vi "LoadGame.vi"(8 "error in (no error)":errorcluster, 10 "NewGame":refnum<class "Game.lvclass">, 11 "Engine in":refnum<class "Engine.lvclass">) -> (0 "error out":errorcluster, 3 "Engine out":refnum<class "Engine.lvclass">)   [LabVIEW 2019, in "RT_Game.lvlib" / "Engine.lvclass"]
uses:
  Engine.lvclass
  Game/Game.lvclass
  Engine.lvclass/Engine.ctl
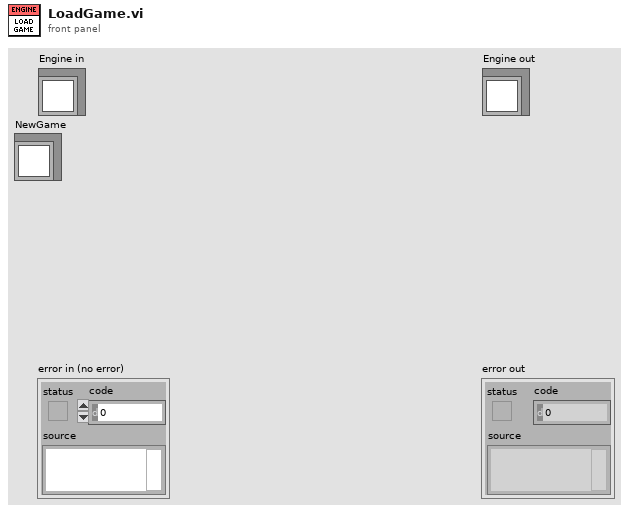
[diagram p1: front panel]
types:
  T1 = typedef "FPGA_Interface.ctl" = refnum<k20>
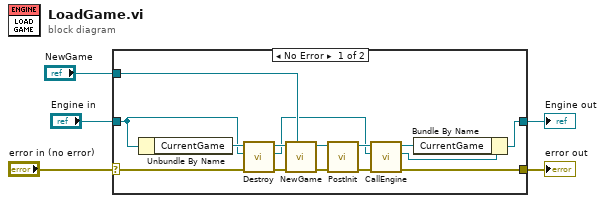
[diagram p0: block diagram]
diagram:
  n1 = case shown="No Error" "error in (no error)" {
    selector: "error in (no error)" -> [w20 w22]
    tunnel: [w11 w22] -> w4
    tunnel: [w19 w21] -> w2
    tunnel: "Engine in" -> [w6 w21]
    tunnel: "NewGame" -> [w17 _]
    frame No Error {
      n2 = Unbundle By Name(w6) -> ("CurrentGame"=w15:refnum<class "Game.lvclass">)
      n3 = call-dynamic "Destroy.vi"("error in (no error)"=w20, "RT_Game.lvlib:Engine.lvclass"=w6, "Game in"=w15) -> ("error out"=w16:errorcluster, "RT_Game.lvlib:Engine.lvclass 2"=w7:refnum<class "Engine.lvclass">, "FPGA_ref"=w14:T1)  [unwired: 6 in]
      n4 = call-dynamic "NewGame.vi"("GameType (ChildObject)"=w17, "error in (no error)"=w16, "FPGA_ref"=w14) -> ("error out"=w18:errorcluster, "Game out"=w12:refnum<class "Game.lvclass">)  [unwired: 7 in]
      n5 = call "PostInit.vi"("error in (no error)"=w18, "Game in"=w12) -> ("error out"=w13:errorcluster, "Game out"=w10:refnum<class "Game.lvclass">)  [unwired: 8 in]
      n6 = call-dynamic "CallEngine.vi"("error in (no error)"=w13, "RT_Game.lvlib:Engine.lvclass"=w7, "Game in"=w10) -> ("error out"=w11:errorcluster, "RT_Game.lvlib:Engine.lvclass 2"=w8:refnum<class "Engine.lvclass">, "Game out"=w9:refnum<class "Game.lvclass">)  [unwired: 6 in]
      n7 = Bundle By Name(cluster=w8, "CurrentGame"=w9) -> (w19:refnum<class "Engine.lvclass">)
    }
    frame Error {
    }
  }
  "error out" <- w4
  "Engine out" <- w2
